vi "多值数值控件.vi"() -> ()   [LabVIEW 2012]
panel:
  out "量表数组":cluster{dbl, dbl, dbl}[](array[knob])=[{0.0, 82.80139732155845, 36.363604693649236}, {0.0, 87.00473479344983, 0.0}, {0.0, 87.00473479344983, 0.0}, {0.0, 87.00473479344983, 0.0}, {0.0, 87.00473479344983, 30.871376692393298}] scale=0.0..100.0
  in  "滑动杆":cluster{dbl, dbl, dbl}(slide)={20.666666666666664, 50.0, 75.51020408163265} scale=0.0..100.0
  out "量表":cluster{dbl, dbl, dbl}(knob)={50.3869201848227, 90.2761129252533, 9.72383880826518} scale=0.0..100.0
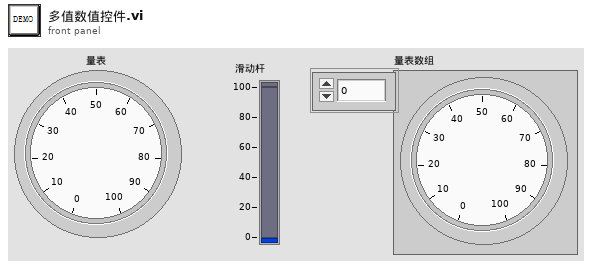
[diagram p1: front panel]
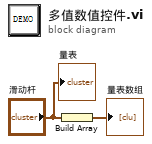
[diagram p0: block diagram]
diagram:
  n1 = Build Array("滑动杆") -> (→"量表数组":cluster{dbl, dbl, dbl}[])
  "量表" <- "滑动杆"
